vi "Merc Gen SCPI Command TCP-IP VI.vi"(2 "error in (no error)":errorcluster, 3 "Command String":string="READ:SYS:CAT", 4 "IP Address":string="172.16.131.11") -> (0 "error out":errorcluster, 1 "read data":string)   [LabVIEW 2013, in "Mercury iXX.lvlib"]
uses:
  Mercury iXX.lvlib
panel:
  out "return count":u32
  # "READ:DEV:DB8.P1:PRES:LOOP"
  # "Note about command strings.\nCommand strings are made up of nouns or verbs separated by colons.\nThe verb is either READ to get a parameter value from the instrument\nor SET to write a parameter value to the instrument.\n\nThis is followed by a noun to define whetner the command is being addressed\nto the system SYS or one of the units devices DEV.  For example to read the\nsystems time the command would be:-\nREAD:SYS:TIME\n\nWhen reading from a device the unique identity (UID) must be supplied as the\nunit may contain many devices.  The UID is a construct of motherboard, MB,\nor daughter board, DB, tag, an index number 0-8, a type letter and index\nand a type (e.g. HTR forheater).  So an example UID would be:-\nMB1.T1.TEMP which represents the index 1 device of the motherboard which\nis a temperature sensor device.\nFor a heater daughter board the UID might be:-\nDB2.H1.HTR where the 2 after DB is the slot number the daughter board is in.\nTo find out what devices are in the unit send the system catalogue command:-\nREAD:SYS:CAT.\n\nFollowing the UID is the actual command.  So to read the voltage signal from\nthe motherboard temperature reading circuit device the command would be:-\nREAD:DEV:MB1.T1:TEMP:SIG:VOLT\nthe reponse should be: -\nSTAT:DEV:MB1.T1:TEMP:SIG:VOLT:11.2345mV\n\nAs an example, to set the voltage limit (VLIM) of the mother board heater output\ncircuit device to 20 volts, the command would be:-\nSET:DEV:MB0.H1:HTR:VLIM:20\nIf successful the response would be:-\nSTAT:SET:DEV:MB0.H1:HTR:VLIM:20:VALID\nIf unsuccessful a response of the form:-\nSTAT:SET:DEV:MB0.H1:HTR:VLIM:20:INVALID\nThe word INVALID will appear directly following the item in the command that the  unit doesn't understand."
  # "SET:DEV:MB1.T1:TEMP:LOOP:RENA:OFF"
  # "SET:DEV:DB8.P1:PRES:LOOP:PRST:500"
  # "SET:DEV:MB1.T1:TEMP:CAL:CAL"
  # "SET:DEV:MB1.T1:TEMP:LOOP:TSET:294.9"
  # "SET:DEV:GRPZ:PSU:VLIM:5.0"
  # "SET:SYS:USER:ENG:abc123"
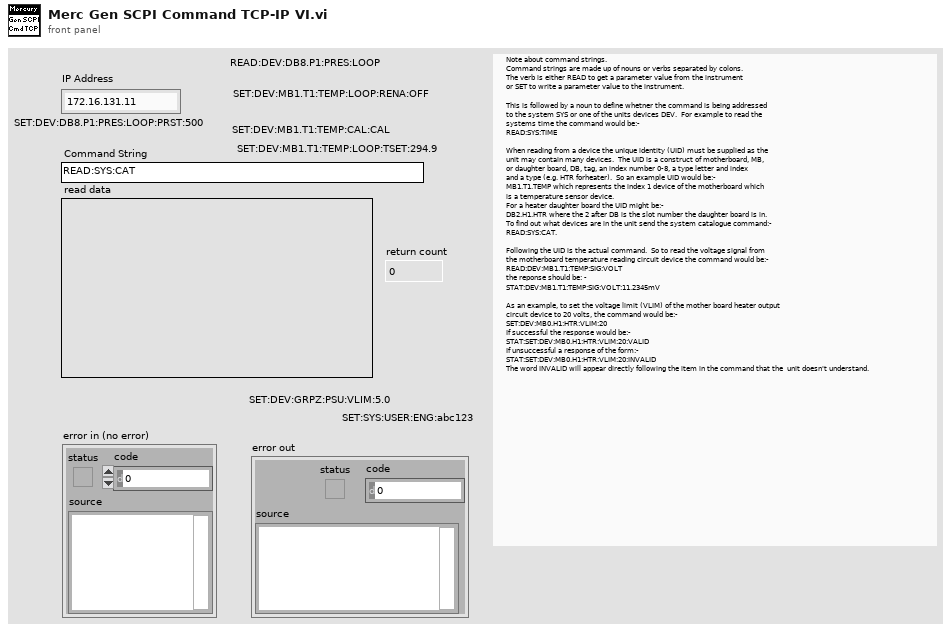
[diagram p1: front panel]
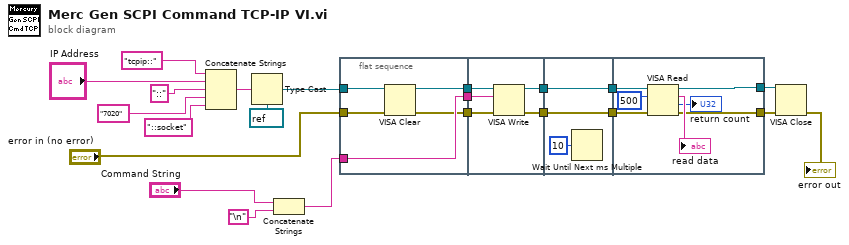
[diagram p0: block diagram]
diagram:
  n1 = Concatenate Strings("tcpip::" ("string"), "IP Address", "::" ("string"), "7020" ("string"), "::socket" ("string")) -> (w12:string)
  n2 = Type Cast(type=refnum<visa-resource-name> refnum ("VISA resource name"), x=w12) -> (*(type *) &x=w4:refnum<visa-resource-name>)
  n3 = Concatenate Strings("Command String", "\n") -> (w7:string)
  n4 = flat-sequence {
    tunnel: "error in (no error)" -> [w25]
    tunnel: w7 -> [w27]
    tunnel: [w26] -> w20
    tunnel: [w27] -> w19
    tunnel: [w24] -> w18
    tunnel: w4 -> [w23]
    tunnel: [w30] -> w17
    tunnel: [w29] -> w16
    tunnel: w20 -> [w32]
    tunnel: w19 -> [w31]
    tunnel: w18 -> [w28]
    tunnel: [w35] -> w15
    tunnel: w17 -> [w35]
    tunnel: w16 -> [w34]
    tunnel: [w34] -> w14
    tunnel: w15 -> [w40]
    tunnel: w14 -> [w39]
    tunnel: [w38] -> w2
    tunnel: [w37] -> w3
    frame #0 {
      n5 = VISA Clear(VISA resource name=w23, error in (no error)=w25) -> (VISA resource name out=w26:refnum<visa-resource-name>, error out=w24:errorcluster)
    }
    frame #1 {
      n6 = VISA Write(VISA resource name=w32, write buffer=w31, error in (no error)=w28) -> (VISA resource name out=w30:refnum<visa-resource-name>, error out=w29:errorcluster)  [unwired: 1 out]
    }
    frame #2 {
      n7 = Wait Until Next ms Multiple(millisecond multiple=u32 10) -> ()  [unwired: 1 out]
    }
    frame #3 {
      n8 = VISA Read(VISA resource name=w40, byte count=u32 500, error in (no error)=w39) -> (VISA resource name out=w37:refnum<visa-resource-name>, read buffer=→"read data":string, return count=→"return count":u32, error out=w38:errorcluster)
    }
  }
  n9 = VISA Close(VISA resource name=w3, error in (no error)=w2) -> (error out=→"error out":errorcluster)
